vi "Dymin_RT_Main.vi"() -> ()   [LabVIEW 2016]
doc: "The myRIO Custom FPGA Project template acquires button data from the onboard button and displays the button value on a Boolean indicator. The SYS.RDY indicator shows the FPGA status."
uses:
  <vilib>/Platform/TimedLoop/XDataNode/timing_clust.ctl
  <vilib>/Platform/TimedLoop/XDataNode/nitl_modes.ctl
  <vilib>/Platform/TimedLoop/XDataNode/wakeup.ctl
  <vilib>/myRIO/Common/Instrument Driver Framework/myRIO v1.0/UART/vis/myRIO v1.0 Close UART.vi
  <vilib>/FPGAPlugInAG/myRIO-1900/niLvFpga_Open_myRIO-1900.vi
  <vilib>/rvi/interface/common/niFpgaWaitOnOcc.vi
  <vilib>/Utility/error.llb/Error Cluster From Error Code.vi
  <vilib>/FPGAPlugInAG/myRIO-1900/niLvFpga_Reset_myRIO-1900.vi
  <vilib>/FPGAPlugInAG/myRIO-1900/niLvFpga_Run_myRIO-1900.vi
  <vilib>/rvi/errors/niLvFpgaAdjustHostInterfaceError.vi
  <vilib>/FPGAPlugInAG/myRIO-1900/niLvFpga_Close_myRIO-1900.vi
  <vilib>/myRIO/Common/Instrument Driver Framework/Utilities/vis/FPGA Ref Manager.vi
  <vilib>/myRIO/Common/Instrument Driver Framework/myRIO v1.0/myRIO v1.0 Reset FPGA.vi
  <vilib>/myRIO/Common/Instrument Driver Framework/myRIO v1.0/IRQ/vis/myRIO v1.0 IRQ Info FGV.vi
  <vilib>/myRIO/Common/Instrument Driver Framework/myRIO v1.0/IRQ/vis/myRIO v1.0 Timer IRQ Info FGV.vi
  <vilib>/myRIO/Common/Instrument Driver Framework/myRIO v1.0/IRQ/vis/myRIO v1.0 ISR Agent.vi
  <vilib>/rvi/interface/nirviOpenFPGA/nirviOpenFPGA.xnode
  FPGA reference.ctl
  FPGA Bitfiles/Dymin4ALL_FPGATarget_FPGAMain_ylQ-wBvMF5Y.lvbitx
  FPGA Main.vi
  <vilib>/rvi/interface/nirviMethod/nirviMethod.xnode
  <vilib>/Platform/TimedLoop/XDataNode/XDataNode.xnode
  <vilib>/rvi/interface/nirviCloseFPGA/nirviCloseFPGA.xnode
  <vilib>/myRIO/Instrument Drivers/Utilities/Utilities.lvlib
  <vilib>/rvi/errors/niLvFpgaMergeErrorWithErrorCode.vi
  <vilib>/Platform/TimedLoop/XDataNode/XDNodeRunTimeDep.lvlib
  <vilib>/FPGAPlugInAG/myRIO-1900/niLvFpga_ConfigureFifo_myRIO-1900.vi
  <vilib>/FPGAPlugInAG/myRIO-1900/niLvFpga_ReadFifo_myRIO-1900.vi
panel:
  out "Throw away Data":u64[](array[numeric])
  in  "stop":bool
  in  "Requested Depth":u32=10000
  out "error out":errorcluster
  # "AOM Voltages:\nIN0=A/AO0\nIN1=C/AO1\nIN2=C/AO0\nIN3=A/AO0\n\nVoltage conversion (raw voltages from FPGA):\nMSP Connectors:\nVoltage=RawDataValue*4.883 mV\nMXP Connectors:\nVoltage=RawDataValue*1.221 mV\nMeasured with 50Ohm\nVoltage=RawDataValue*2.1mV\n\nI have calibrated the program to the voltage output into 50 Ohms, you will need to calibrate it to your system."
  # "Requirements: \nLabview 2016 (32 bit)\nLabview Real-Time Module\nLabview FPGA Module\nCompile Cloud access (Sign up at https://www.ni.com/en-us/support/documentation/supplemental/14/compile-faster-with-the-labview-fpga-compile-cloud-service.html)\nOR Xilinx Compilation Tools to compile the code on your FPGA.\n.\nInstructions:\n1. Check the myRIO target IP address in the project and make sure the target IP address is correct. \n2. Run this VI."
  # "Size of time bits\n1 bit=12.5 ns"
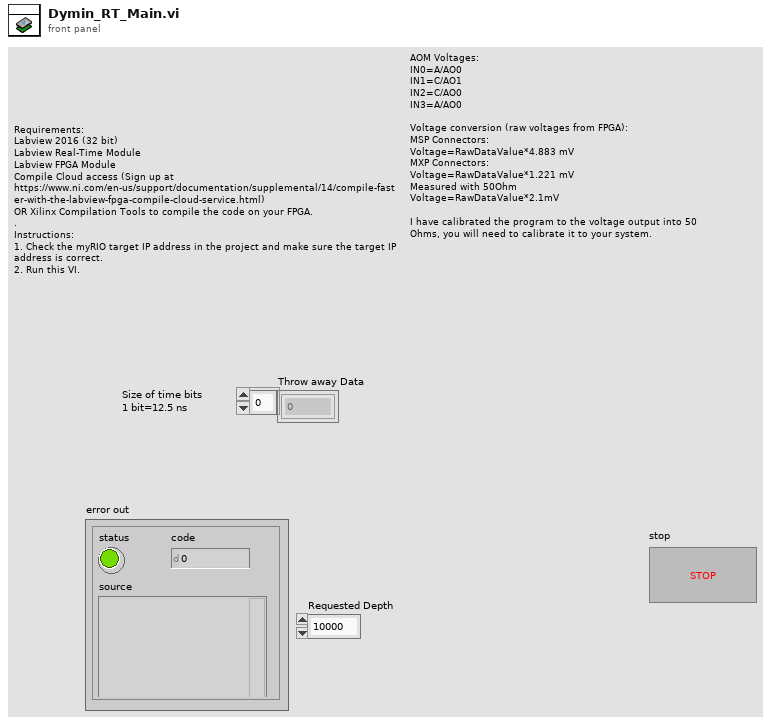
[diagram p1: front panel]
types:
  T1 = typedef "XDNodeRunTimeDep.lvlib/timing_clust.ctl" = cluster{"Expected End [f-1]":u64, "Actual End [f-1]":u64, "Finished Late? [f-1]":bool, "Expected End [i-1]":u64, "Actual End [i-1]":u64, "Finished Late? [i-1]":bool, "Expected Start [i]":u64, "Actual Start [i]":u64, "Expected Start [f]":u64, "Actual Start [f]":u64, "Source Name":string, "Structure Name":string, "Period":i64, "Deadline":i64, "Offset":i64, "Start":i64, "Priority":i32, "Timeout":i32, "Mode":T2, "Wakeup Reason":T3, "Error":errorcluster, "Source Type":string, "Secondary Source Type":string, "Global End Time":u64, "Global Start Time":u64, "Frame Duration":u64, "Iteration Duration":u64, "Assigned CPU":i32, "I/O Scan Engine Mode":u32}
  T2 = typedef "XDNodeRunTimeDep.lvlib/nitl_modes.ctl" = enum32{"No Change", "Process missed periods, maintain original phase", "Discard missed periods, maintain original phase", "Process missed periods, ignore original phase", "Discard missed periods, ignore original phase"}
  T3 = typedef "XDNodeRunTimeDep.lvlib/wakeup.ctl" = enum32{"Normal", "Aborted", "Asynchronous wakeup", "Timing source error", "Timed loop error", "Timeout"}
  T4 = typedef "FPGA reference.ctl" = refnum<k20>
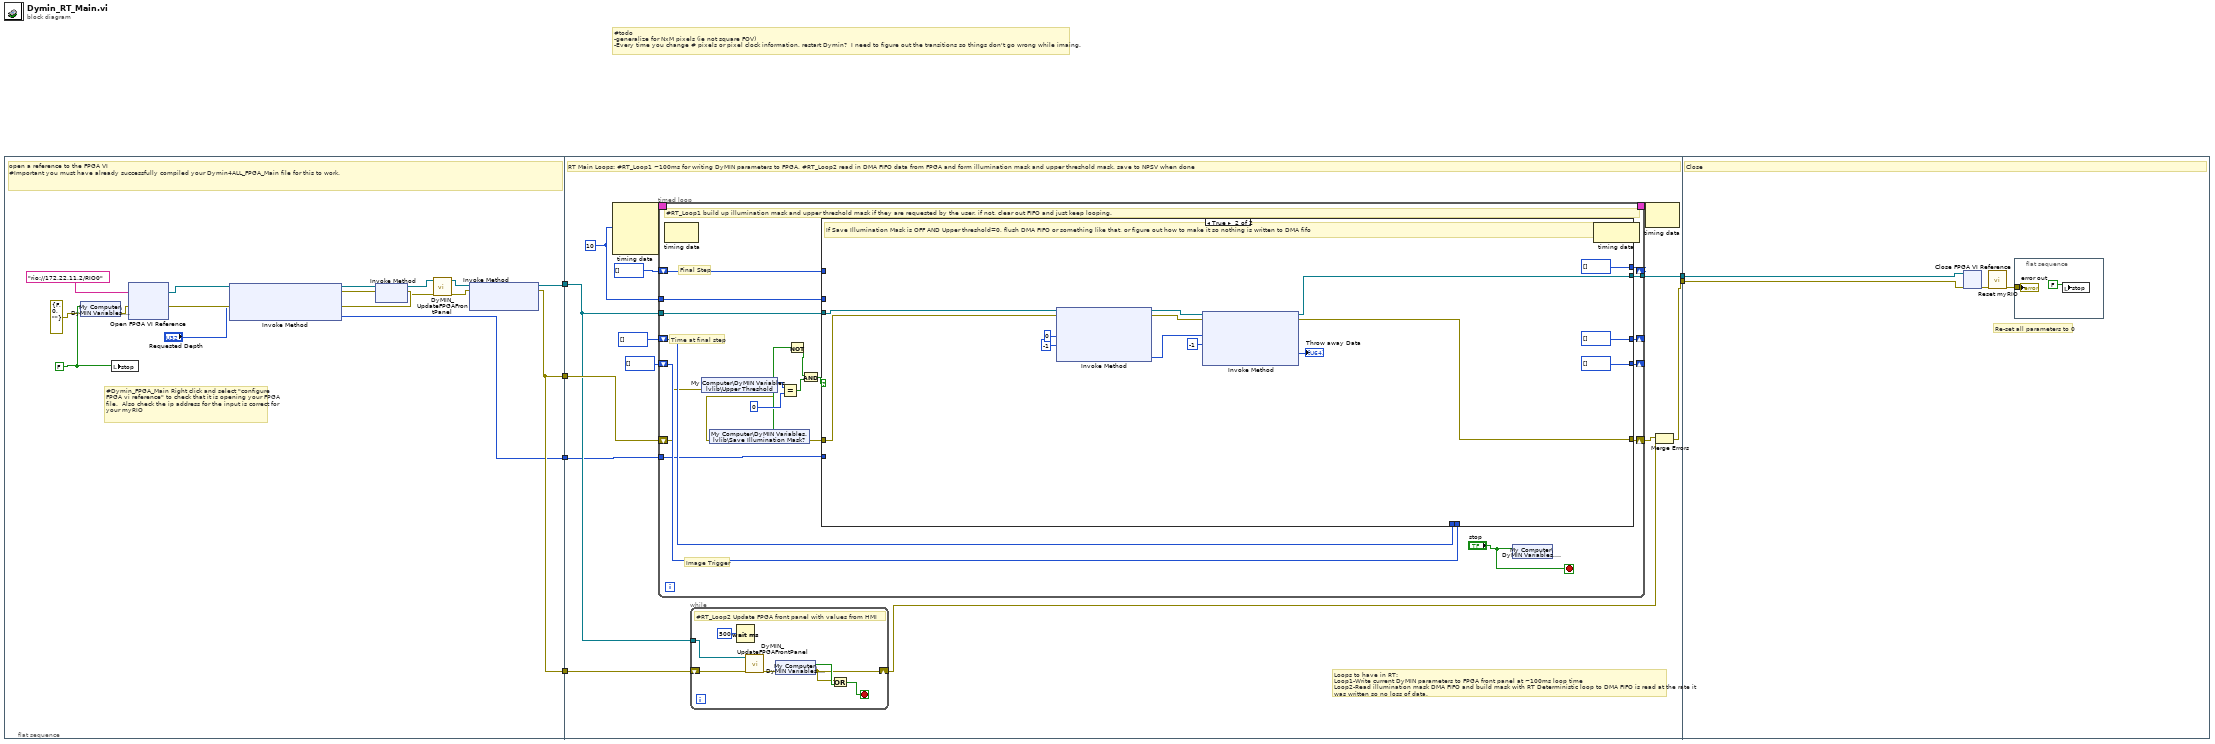
[diagram p0: block diagram]
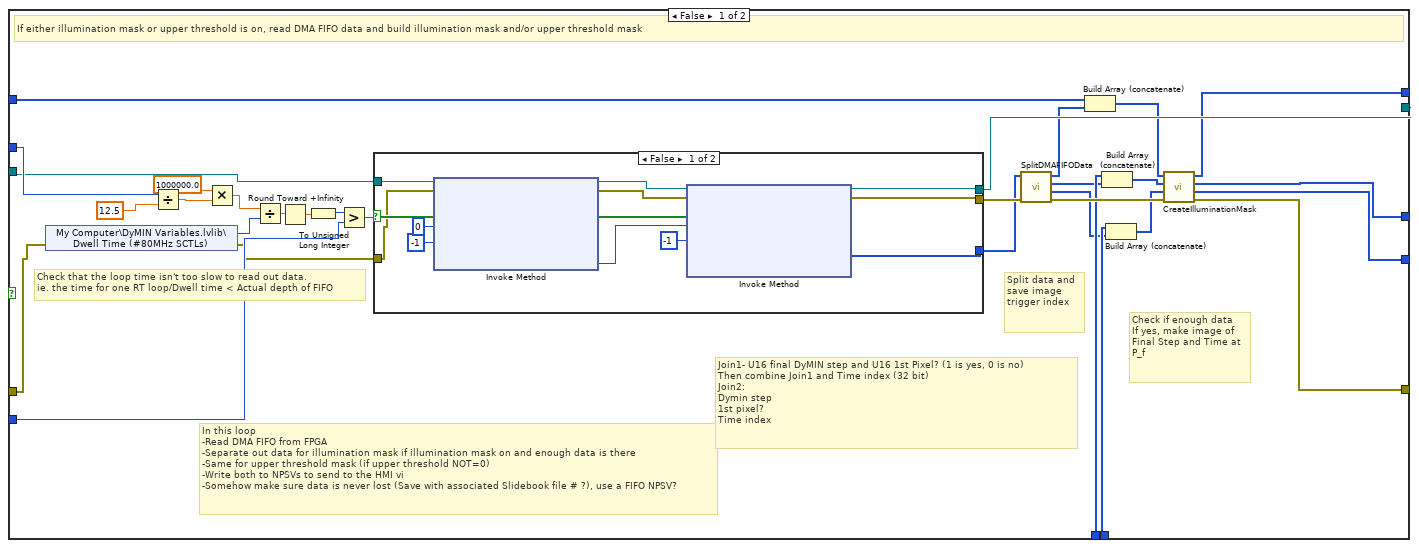
[diagram p2: hidden frame]
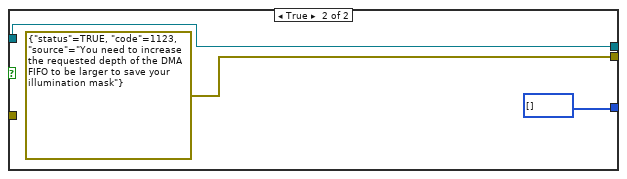
[diagram p3: hidden frame]
diagram:
  # "#todo\n-generalize for NxM pixels (ie not square FOV)\n-Every time you change # pixels or pixel clock information, restart Dymin?  I need to figure out the transitions so things don't go wrong while imaing."
  n1 = flat-sequence {
    tunnel: [w17] -> w5
    tunnel: [w18] -> w4
    tunnel: [w17] -> w2
    tunnel: [w7] -> w1
    tunnel: [w23] -> w6
    tunnel: w5 -> [w36]
    tunnel: w4 -> [w27]
    tunnel: [w35] -> w3
    tunnel: w2 -> [w31]
    tunnel: w1 -> [w26]
    tunnel: w6 -> [w133]
    tunnel: w3 -> [w130]
    frame #0 {
      w16 = FALSE ("Stop")
      # "#Dymin_FPGA_Main Right click and select \"configure FPGA vi reference\" to check that it is opening your FPGA file.  Also check the ip address for the input is correct for your myRIO"
      # "open a reference to the FPGA VI\n#Important you must have already successfully compiled your Dymin4ALL_FPGA_Main file for this to work."
      n2 = shared-variable "My Computer\\DyMIN Variables.lvlib\\Stop"(w16, error in=errorcluster {"status"=FALSE, "code"=0, "source"=""}) -> (error out=w8:errorcluster)
      n3 = local write "stop"(w16) -> ()
      n4 = xnode "Open FPGA VI Reference"("error in"=w8, "resource name"=tag "rio://172.22.11.2/RIO0") -> ("FPGA VI Reference Out"=w14:T4, "error out"=w21:errorcluster)
      n5 = xnode "Invoke Method"("FPGA VI Reference In"=w14, "error in"=w21, "Requested Depth"="Requested Depth") -> ("FPGA VI Reference Out"=w19:T4, "error out"=w15:errorcluster, "Actual Depth"=w7:u32)
      n6 = xnode "Invoke Method"("FPGA VI Reference In"=w19, "error in"=w15) -> ("FPGA VI Reference Out"=w12:T4, "error out"=w11:errorcluster)
      n7 = call "DyMIN_UpdateFPGAFrontPanel.vi"("error in (no error)"=w11, "FPGA Ref IN"=w12) -> ("error out"=w9:errorcluster, "FPGA Ref OUT"=w10:T4)  [unwired: 8 in]
      n8 = xnode "Invoke Method"("FPGA VI Reference In"=w10, "error in"=w9) -> ("FPGA VI Reference Out"=w18:T4, "error out"=w17:errorcluster)  [unwired: 1 in]
    }
    frame #1 {
      w28 = i64 10 ("Period")
      # "Loops to have in RT:\nLoop1-Write current DyMIN parameters to FPGA front panel at ~100ms loop time\nLoop2-Read illumination mask DMA FIFO and build mask with RT Deterministic loop to DMA FIFO is read at the rate it was written so no loss of data."
      # "RT Main Loops: #RT_Loop1 ~100ms for writing DyMIN parameters to FPGA, #RT_Loop2 read in DMA FIFO data from FPGA and form illumination mask and upper threshold mask, save to NPSV when done"
      n9 = node-c288(w28) -> (w30:T1)  [unwired: 3 in]
      n10 = timed-loop {
        tunnel: w27 -> [w47]
        shift-right: [w42] -> w24
        shift-left: w36 -> [w38]
        tunnel: [w57] -> w35
        shift-right: [w41] -> _
        shift-left: u16[] [] -> [w56]
        shift-right: [w46] -> _
        shift-left: u16[] [] -> [w48]
        shift-right: [w43] -> _
        shift-left: u32[] [] -> [w45]
        timing: w30 -> [_]
        timing-out: [_] -> w29
        tunnel: w28 -> [w49]
        tunnel: w26 -> [w40]
        stop <- "stop" stop-if-true
        # "Final Step"
        # "Time at final step"
        # "Image Trigger"
        # "#RT_Loop1 build up illumination mask and upper threshold mask if they are requested by the user, if not, clear out FIFO and just keep looping."
        n11 = node-c288() -> ()  [unwired: 1 in, 1 out]
        n12 = shared-variable "My Computer\\DyMIN Variables.lvlib\\Upper Threshold"(error in=w38) -> (w55:u32, error out=w37:errorcluster)
        n13 = shared-variable "My Computer\\DyMIN Variables.lvlib\\Save Illumination Mask?"(error in=w37) -> (w53:bool, error out=w39:errorcluster)
        n14 = Equal?(x=w55, y=u32 0) -> (x = y?=w51:bool)
        n15 = Not(x=w53) -> (.not. x?=w52:bool)
        n16 = And(x=w52, y=w51) -> (x .and. y?=w50:bool)
        n17 = case shown="True" w50 {
          tunnel: [w89 w111] -> w57
          tunnel: w45 -> [w83 _]
          tunnel: w56 -> [w82 _]
          tunnel: w49 -> [w79 _]
          tunnel: w48 -> [w74 _]
          tunnel: w47 -> [w73 w113]
          tunnel: [w66 u16[] [] ("Final step OUT")] -> w46
          tunnel: [w64 u16[] [] ("Image trig OUT")] -> w41
          tunnel: [w65 u32[] [] ("Time at P_f OUT")] -> w43
          tunnel: [w63 w108] -> w42
          tunnel: w39 -> [w61 w109]
          tunnel: w40 -> [w62 _]
          frame False {
            # "Check that the loop time isn't too slow to read out data.\nie. the time for one RT loop/Dwell time < Actual depth of FIFO"
            # "In this loop\n-Read DMA FIFO from FPGA\n-Separate out data for illumination mask if illumination mask on and enough data is there\n-Same for upper threshold mask (if upper threshold NOT=0)\n-Write both to NPSVs to send to the HMI vi\n-Somehow make sure data is never lost (Save with associated Slidebook file # ?), use a FIFO NPSV?"
            # "Check if enough data\nIf yes, make image of Final Step and Time at P_f"
            # "Split data and save image trigger index"
            # "Join1- U16 final DyMIN step and U16 1st Pixel? (1 is yes, 0 is no)\nThen combine Join1 and Time index (32 bit)\nJoin2:\nDymin step\n1st pixel?\nTime index"
            # "If either illumination mask or upper threshold is on, read DMA FIFO data and build illumination mask and/or upper threshold mask"
            n18 = shared-variable "My Computer\\DyMIN Variables.lvlib\\Dwell Time (#80MHz SCTLs)"(error in=w61) -> (w80:u32, error out=w60:errorcluster)
            n19 = Divide(x=w79, y=12.5) -> (x/y=w77:dbl)
            n20 = Multiply(x=1000000.0, y=w77) -> (x*y=w75:dbl)
            n21 = Divide(x=w75, y=w80) -> (x/y=w72:dbl)
            n22 = Round Toward +Infinity(x=w72) -> (ceil(x): smallest int >= x=w71:dbl)
            n23 = To Unsigned Long Integer(number=w71) -> (unsigned 32bit integer=w88:u32)
            n24 = Greater?(x=w88, y=w62) -> (0:w90:bool)
            n25 = case shown="False" w90 {
              tunnel: [w98 w102] -> w89
              tunnel: [w94 errorcluster {"status"=TRUE, "code"=1123, "source"="You need to increase the requested depth of the DMA FIFO to be larger to save your illumination mask"} ("error in")] -> w87
              tunnel: [w95 u64[] [] ("Data")] -> w85
              tunnel: w73 -> [w93 w102]
              tunnel: w60 -> [w92 _]
              frame False {
                n26 = xnode "Invoke Method"("FPGA VI Reference In"=w93, "error in"=w92, "Number of Elements"=u32 0, "Timeout (ms)"=-1) -> ("FPGA VI Reference Out"=w91:T4, "error out"=w99:errorcluster, "Elements Remaining"=w97:u32)  [unwired: 1 out]
                n27 = xnode "Invoke Method"("FPGA VI Reference In"=w91, "error in"=w99, "Number of Elements"=w97, "Timeout (ms)"=-1) -> ("FPGA VI Reference Out"=w98:T4, "error out"=w94:errorcluster, "Data"=w95:u64[])  [unwired: 1 out]
              }
              frame True {
              }
            }
            n28 = call "SplitDMAFIFOData.vi"("error in (no error)"=w87, "Data Array IN"=w85) -> ("error out"=w86:errorcluster, "Image trig"=w81:u16[], "Time at P_final if less than t_final"=w69:u32[], "Final step, n"=w84:u16[])  [unwired: 6 in]
            n29 = Build Array (concatenate)(w74, w84) -> (w70:u16[])
            n30 = Build Array (concatenate)(w83, w69) -> (w68:u32[])
            n31 = Build Array (concatenate)(w82, w81) -> (w67:u16[])
            n32 = call "CreateIlluminationMask.vi"("error in (no error)"=w86, "Image trig"=w67, "Time at P_f"=w68, "Final step, n"=w70) -> ("error out"=w63:errorcluster, "Image trig OUT"=w64:u16[], "Time at P_f OUT"=w65:u32[], "Final step OUT"=w66:u16[])  [unwired: 4 in]
          }
          frame True {
            # "If Save Illumination Mask is OFF AND Upper threshold=0, flush DMA FIFO or something like that, or figure out how to make it so nothing is written to DMA fifo"
            n33 = xnode "Invoke Method"("FPGA VI Reference In"=w113, "error in"=w109, "Number of Elements"=u32 0, "Timeout (ms)"=-1) -> ("FPGA VI Reference Out"=w112:T4, "error out"=w116:errorcluster, "Elements Remaining"=w115:u32)  [unwired: 1 out]
            n34 = xnode "Invoke Method"("FPGA VI Reference In"=w112, "error in"=w116, "Number of Elements"=w115, "Timeout (ms)"=-1) -> ("FPGA VI Reference Out"=w111:T4, "error out"=w108:errorcluster, "Data"=→"Throw away Data":u64[])  [unwired: 1 out]
          }
        }
        n35 = shared-variable "My Computer\\DyMIN Variables.lvlib\\Stop"("stop") -> ()  [unwired: 1 in, 1 out]
        n36 = node-c288() -> ()  [unwired: 1 in, 1 out]
      }
      n37 = while {
        shift-right: [w126] -> w25
        shift-left: w31 -> [w124]
        tunnel: w27 -> [w125]
        stop <- w128 stop-if-true
        # "#RT_Loop2 Update FPGA front panel with values from HMI"
        n38 = Wait (ms)(milliseconds to wait=u32 500) -> ()  [unwired: 1 out]
        n39 = call "DyMIN_UpdateFPGAFrontPanel.vi"("error in (no error)"=w124, "FPGA Ref IN"=w125) -> ("error out"=w123:errorcluster)  [unwired: 8 in, 1 out]
        n40 = shared-variable "My Computer\\DyMIN Variables.lvlib\\Stop"(error in=w123) -> (w127:bool, error out=w126:errorcluster)
        n41 = Or(x=w126, y=w127) -> (x .or. y?=w128:bool)
      }
      n42 = node-c288(w29) -> ()  [unwired: 1 out]
      n43 = Merge Errors(w24, w25) -> (w23:errorcluster)
    }
    frame #2 {
      # "Re-set all parameters to 0"
      # "Close"
      n44 = xnode "Close FPGA VI Reference"("FPGA VI Reference In"=w130, "error in"=w133) -> ("error out"=w132:errorcluster)
      n45 = call <vilib>:"Reset myRIO.vi"("error in (no error)"=w132) -> ("error out"=w131:errorcluster)  [unwired: 10 in]
      n46 = flat-sequence {
        tunnel: w131 -> [w135]
        frame #0 {
          n47 = local write "stop"(FALSE ("stop")) -> ()
          "error out" <- w135
        }
      }
    }
  }
